vi "Compile Knock Sensor 1.0 Data.vi"(8 "error in (no error)":errorcluster, 11 "Device Item Ref in":T3 format="%.0x") -> (0 "error out":errorcluster, 2 "Knock Sensors":T1[](array[typedef]), 3 "Device Item Ref out":T3 format="%.0x")   [LabVIEW 2013, in "Engine Simulation Toolkit System Explorer.lvlib"]
uses:
  Engine Simulation Toolkit System Explorer.lvlib
  <vilib>/NI Veristand/Custom Device API/Custom Device Item Ref.ctl
  Shared/1.0 Knock Sensor Engine Data.ctl
  Shared/1.0 Knock Sensor FIFO Idxs.ctl
  Knock Low Freq Setting.ctl
  Shared/Constants and GUIDs.vi
  <vilib>/NI Veristand/Custom Device Tools/Custom Device Utility Library/NI VeriStand - Search for All Items by GUID.vi
  Shared/Properties.vi
  <vilib>/NI Veristand/Custom Device API/Get Item Property (String).vi
  <vilib>/NI Veristand/Custom Device API/Get Item Property (U16).vi
  <vilib>/NI Veristand/Custom Device API/Get Item Property (Double).vi
  Shared/Engine Simulation Toolkit Shared.lvlib
  <vilib>/NI Veristand/Custom Device Tools/Custom Device Utility Library/Custom Device Utility Library.lvlib
  <vilib>/NI Veristand/Custom Device API/Custom Device API.lvlib
  <vilib>/rvi/Analysis/host/Public/NI_FpgaMspHost.lvlib
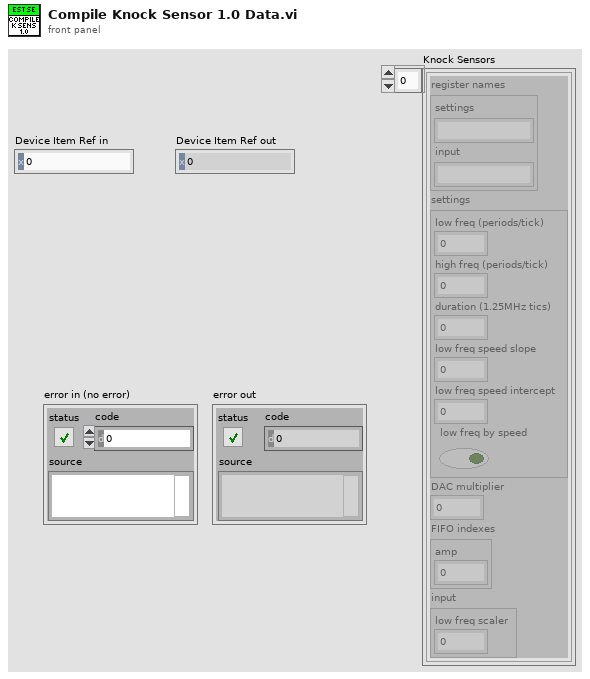
[diagram p1: front panel]
types:
  T1 = typedef "Engine Simulation Toolkit Shared.lvlib/1.0 Knock Sensor Engine Data.ctl" = cluster{"register names":cluster{"settings":string, "input":string}, "settings":cluster{"low freq (periods/tick)":fxp<+,32,0>, "high freq (periods/tick)":fxp<+,32,0>, "duration (1.25MHz tics)":fxp<+,18,18>, "low freq speed slope":fxp<+,16,-3>, "low freq speed intercept":fxp<+,10,-10>, "low freq by speed":bool}, "DAC multiplier":dbl, "FIFO indexes":T2, "input":cluster{"low freq scaler":fxp<+,10,0>}}
  T2 = typedef "Engine Simulation Toolkit Shared.lvlib/1.0 Knock Sensor FIFO Idxs.ctl" = cluster{"amp":i32}
  T3 = typedef "Custom Device API.lvlib/Custom Device Item Ref.ctl" = u64
  T4 = typedef "Engine Simulation Toolkit Shared.lvlib/Channel.ctl" = cluster{"Name":string, "Units":string, "Default":dbl, "Description":string}
  T5 = typedef "Engine Simulation Toolkit System Explorer.lvlib/Knock Low Freq Setting.ctl" = enum16{"Manually", "As function of speed"}
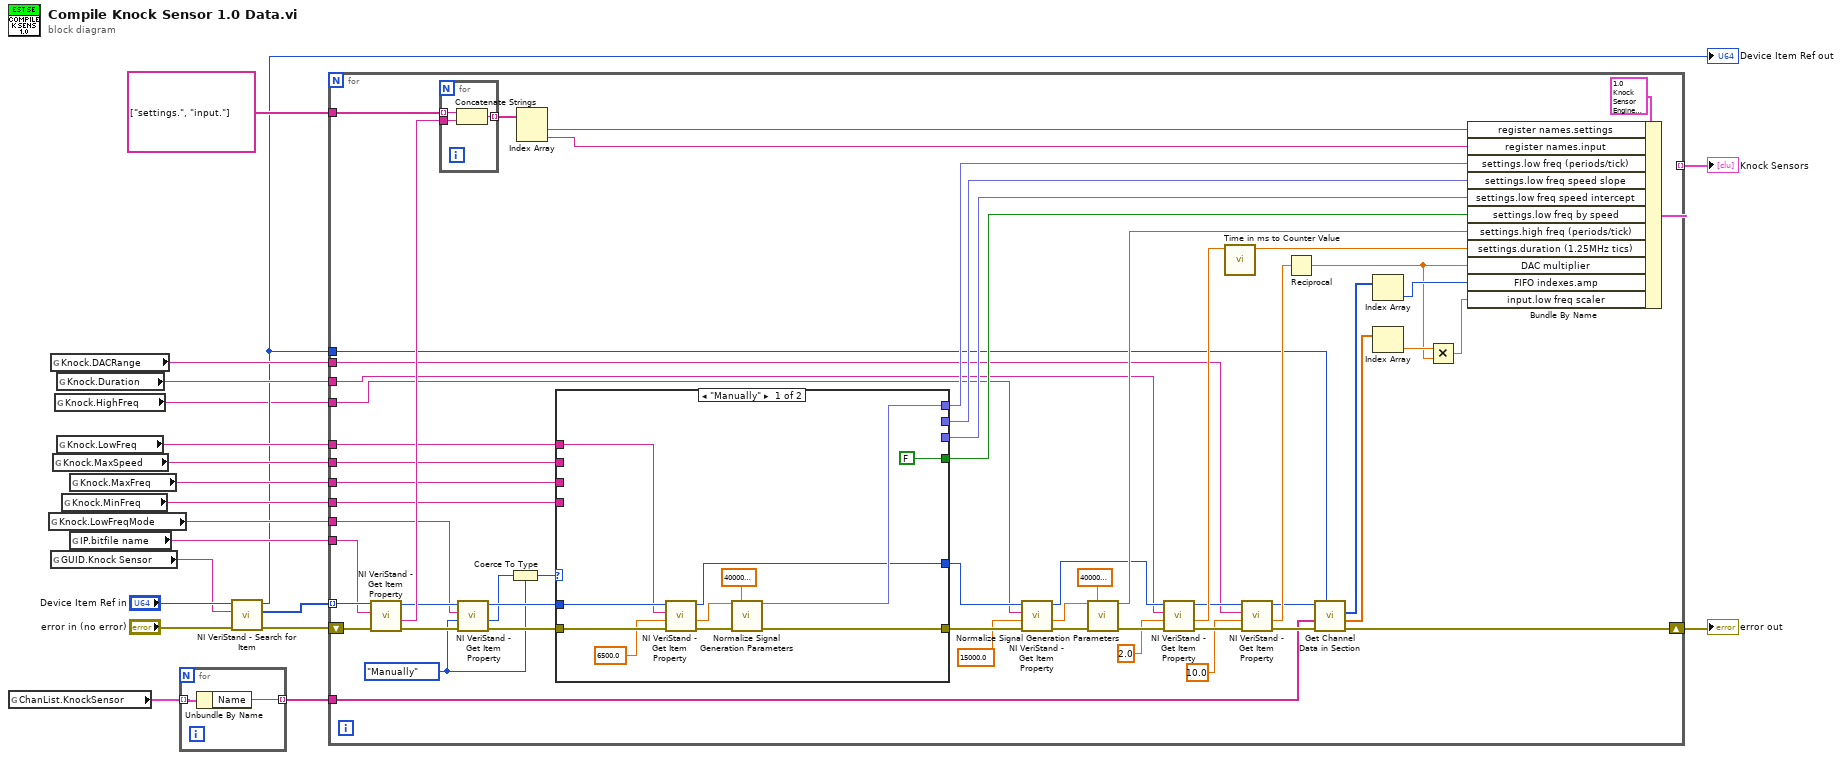
[diagram p0: block diagram]
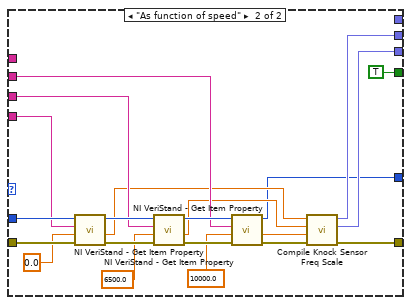
[diagram p2: hidden frame]
diagram:
  n1 = global read "Constants and GUIDs.vi" "ChanList.KnockSensor"() -> (w7:T4[])
  n2 = global read "Properties.vi" "Knock.LowFreqMode"() -> (w11:string)
  n3 = global read "Properties.vi" "Knock.DACRange"() -> (w3:string)
  n4 = global read "Constants and GUIDs.vi" "GUID.Knock Sensor"() -> (w15:string)
  n5 = global read "Properties.vi" "Knock.MaxSpeed"() -> (w8:string)
  n6 = global read "Properties.vi" "Knock.HighFreq"() -> (w1:string)
  n7 = global read "Properties.vi" "Knock.Duration"() -> (w4:string)
  n8 = global read "Properties.vi" "Knock.LowFreq"() -> (w5:string)
  n9 = global read "Properties.vi" "Knock.MinFreq"() -> (w10:string)
  n10 = global read "Properties.vi" "Knock.MaxFreq"() -> (w9:string)
  n11 = global read "Properties.vi" "IP.bitfile name"() -> (w12:string)
  n12 = for {
    tunnel: w7 -> [w22] mode=indexing
    tunnel: [w21] -> w6 mode=indexing
    n13 = Unbundle By Name(w22) -> ("Name"=w21:string)
  }
  n14 = call-poly <vilib>:"NI VeriStand - Search for Item.vi"("error in"="error in (no error)", "Item GUID"=w15, "Section Ref in"="Device Item Ref in") -> ("error out"=w14:errorcluster, "Item Refs"=w13:T3[], "Section Ref out"=w2:T3)  [unwired: 5 in, 1 out]
  "Device Item Ref out" <- w2
  n15 = for {
    shift-right: [w33] -> w17
    shift-left: w14 -> [w74]
    tunnel: string[] ["settings.", "input."] -> [w78]
    tunnel: [w76] -> w16 mode=indexing
    tunnel: w13 -> [w73] mode=indexing
    tunnel: w12 -> [w72]
    tunnel: w11 -> [w65]
    tunnel: w10 -> [w64]
    tunnel: w9 -> [w63]
    tunnel: w8 -> [w62]
    tunnel: w6 -> [w30]
    tunnel: w5 -> [w57]
    tunnel: w4 -> [w42]
    tunnel: w3 -> [w36]
    tunnel: w2 -> [w32]
    tunnel: w1 -> [w23]
    w59 = Knock_Low_Freq_Setting."Manually" ("Low frequency (Hz)")
    n16 = call-poly <vilib>:"NI VeriStand - Get Item Property.vi"("error in (no error)"=w74, "Property Name"=w72, "Item Ref in"=w73) -> ("error out"=w67:errorcluster, "Value"=w71:string, "Item Ref out"=w66:T3)  [unwired: 5 in, 1 out]
    n17 = for {
      tunnel: w78 -> [w113] mode=indexing
      tunnel: [w112] -> w75 mode=indexing
      tunnel: w71 -> [w111]
      n18 = Concatenate Strings(w113, w111) -> (w112:string)
    }
    n19 = call-poly <vilib>:"NI VeriStand - Get Item Property.vi"("error in (no error)"=w67, "Default Value"=w59, "Property Name"=w65, "Item Ref in"=w66) -> ("error out"=w68:errorcluster, "Value"=w60:u16, "Item Ref out"=w69:T3)  [unwired: 4 in, 1 out]
    n20 = Coerce To Type(0:w60, 1:w59) -> (2:w58:T5)
    n21 = Index Array(array=w75) -> (element #1=w70:string, element #2=w61:string)  [unwired: 2 in]
    n22 = case shown="\"Manually\"" w58 {
      tunnel: w69 -> [w87 w108]
      tunnel: w68 -> [w89 w107]
      tunnel: w64 -> [_ w104]
      tunnel: w63 -> [_ w103]
      tunnel: w62 -> [_ w102]
      tunnel: [w84 w100] -> w49
      tunnel: [_ w93] -> w54
      tunnel: [_ w92] -> w53
      tunnel: w57 -> [w86 _]
      tunnel: [w81 _] -> w56
      tunnel: [FALSE ("settings.low freq by speed") TRUE ("settings.low freq by speed")] -> w55
      tunnel: [w79 w90] -> w48
      frame "Manually" {
        n23 = call-poly <vilib>:"NI VeriStand - Get Item Property.vi"("error in (no error)"=w89, "Default Value"=6500.0, "Property Name"=w86, "Item Ref in"=w87) -> ("error out"=w88:errorcluster, "Value"=w83:dbl, "Item Ref out"=w79:T3)  [unwired: 4 in, 1 out]
        n24 = call <vilib>:"Normalize Signal Generation Parameters.vi"("frequency (Hz)"=w83, "FPGA clock rate (Hz)"=40000000.0, "error in (no error)"=w88) -> ("frequency (periods/tick)"=w81:fxp<+,32,0>, "error out"=w84:errorcluster)  [unwired: 7 in, 4 out]
      }
      frame "As function of speed" {
        n25 = call-poly <vilib>:"NI VeriStand - Get Item Property.vi"("error in (no error)"=w107, "Default Value"=0.0, "Property Name"=w104, "Item Ref in"=w108) -> ("error out"=w105:errorcluster, "Value"=w99:dbl, "Item Ref out"=w106:T3)  [unwired: 4 in, 1 out]
        n26 = call-poly <vilib>:"NI VeriStand - Get Item Property.vi"("error in (no error)"=w105, "Default Value"=6500.0, "Property Name"=w103, "Item Ref in"=w106) -> ("error out"=w110:errorcluster, "Value"=w95:dbl, "Item Ref out"=w109:T3)  [unwired: 4 in, 1 out]
        n27 = call-poly <vilib>:"NI VeriStand - Get Item Property.vi"("error in (no error)"=w110, "Default Value"=10000.0, "Property Name"=w102, "Item Ref in"=w109) -> ("error out"=w101:errorcluster, "Value"=w94:dbl, "Item Ref out"=w90:T3)  [unwired: 4 in, 1 out]
        n28 = call "Compile Knock Sensor Freq Scale.vi"("error in (no error)"=w101, "max rpm"=w94, "max freq"=w95, "min freq"=w99) -> ("error out"=w100:errorcluster, "fxp intercept (b)"=w92:fxp<+,10,-10>, "fxp slope (m)"=w93:fxp<+,16,-3>)  [unwired: 5 in]
      }
    }
    n29 = call-poly <vilib>:"NI VeriStand - Get Item Property.vi"("error in (no error)"=w49, "Default Value"=15000.0, "Property Name"=w23, "Item Ref in"=w48) -> ("error out"=w50:errorcluster, "Value"=w51:dbl, "Item Ref out"=w43:T3)  [unwired: 4 in, 1 out]
    n30 = call <vilib>:"Normalize Signal Generation Parameters.vi"("frequency (Hz)"=w51, "FPGA clock rate (Hz)"=40000000.0, "error in (no error)"=w50) -> ("frequency (periods/tick)"=w45:fxp<+,32,0>, "error out"=w46:errorcluster)  [unwired: 7 in, 4 out]
    n31 = call-poly <vilib>:"NI VeriStand - Get Item Property.vi"("error in (no error)"=w46, "Default Value"=2.0, "Property Name"=w42, "Item Ref in"=w43) -> ("error out"=w44:errorcluster, "Value"=w40:dbl, "Item Ref out"=w37:T3)  [unwired: 4 in, 1 out]
    n32 = call "Time in ms to Counter Value.vi"("time (ms)"=w40) -> ("counter value"=w39:dbl)  [unwired: 10 in]
    n33 = call-poly <vilib>:"NI VeriStand - Get Item Property.vi"("error in (no error)"=w44, "Default Value"=10.0, "Property Name"=w36, "Item Ref in"=w37) -> ("error out"=w38:errorcluster, "Value"=w34:dbl, "Item Ref out"=w31:T3)  [unwired: 4 in, 1 out]
    n34 = Reciprocal(x=w34) -> (1/x=w25:dbl)
    n35 = call "Get Channel Data in Section.vi"("Custom device ref"=w32, "error in (no error)"=w38, "Channels"=w30, "Item Ref in"=w31) -> ("error out"=w33:errorcluster, "default values"=w27:dbl[], "FIFO indexes"=w29:i32[])  [unwired: 3 in, 2 out]
    n36 = Index Array(array=w29) -> (element=w28:i32)  [unwired: 1 in]
    n37 = Index Array(array=w27) -> (element=w26:dbl)  [unwired: 1 in]
    n38 = Multiply(x=w26, y=w25) -> (x*y=w24:dbl)
    n39 = Bundle By Name(cluster=T1 {"register names"={"settings"="", "input"=""}, "settings"={"low freq (periods/tick)"=0.0, "high freq (periods/tick)"=0.0, "duration (1.25MHz tics)"=0.0, "low freq speed slope"=0.0, "low freq speed intercept"=0.0, "low freq by speed"=FALSE}, "DAC multiplier"=0.0, "FIFO indexes"={"amp"=0}, "input"={"low freq scaler"=0.0}} ("1.0.0 Knock Sensor"), "register names.settings"=w70, "register names.input"=w61, "settings.low freq (periods/tick)"=w56, "settings.low freq speed slope"=w54, "settings.low freq speed intercept"=w53, "settings.low freq by speed"=w55, "settings.high freq (periods/tick)"=w45, "settings.duration (1.25MHz tics)"=w39, "DAC multiplier"=w25, "FIFO indexes.amp"=w28, "input.low freq scaler"=w24) -> (w76:T1)
  }
  "error out" <- w17
  "Knock Sensors" <- w16
